vi "UTILITY JKI Loop Timer.vi"(7 "Initialize Rate":bool, 9 "Min Setpoint":T1=0.2 format="%.2f", 10 "K(0.3)":dbl=0.3 format="%#_13g", 11 "Scan Rate (Seconds)":dbl) -> (2 "Rate":dbl, 3 "New Time":dbl)   [LabVIEW 2019]
uses:
  Custom Pallet Controls/Custom Pallet DBL.ctl
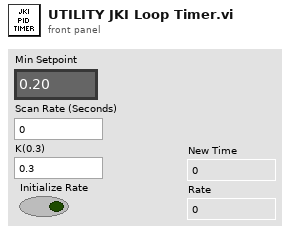
[diagram p1: front panel]
types:
  T1 = typedef "Custom Pallet DBL.ctl" = dbl
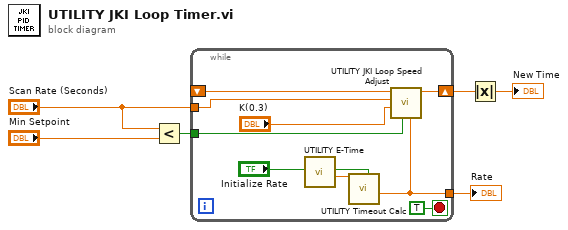
[diagram p0: block diagram]
diagram:
  n1 = Less?(x="Scan Rate (Seconds)", y="Min Setpoint") -> (x < y?=w3:bool)
  n2 = while {
    shift-right: [w10] -> w1
    shift-left: _ -> [w14]
    tunnel: "Scan Rate (Seconds)" -> [w8]
    tunnel: [w9] -> w6
    tunnel: w3 -> [w11]
    stop <- TRUE stop-if-true
    n3 = call "UTILITY E-Time.vi"() -> ("Elapsed Time (sec)"=w15:dbl)  [unwired: 9 in, 2 out]
    n4 = call "UTILITY Timeout Calc.vi"("Initialize Rate"="Initialize Rate", "Timer"=w15) -> ("Rate"=w9:dbl)  [unwired: 8 in, 1 out]
    n5 = call "UTILITY JKI Loop Speed Adjust.vi"("Current Rate"=w9, "Scan Rate Less Than 0.2s"=w11, "K(7) - Adjustment Factor"="K(0.3)", "Scan Rate Target"=w8, "Previous Value"=w14) -> ("New Time"=w10:dbl)  [unwired: 6 in]
  }
  "Rate" <- w6
  n6 = Absolute Value(x=w1) -> (abs(x)=→"New Time":dbl)
